vi "decimateInput.vi"(8 "reset":bool, 9 "input":i16, 10 "zeroOutput":bool, 11 "invert":bool) -> (3 "output":i16)   [LabVIEW 2016]
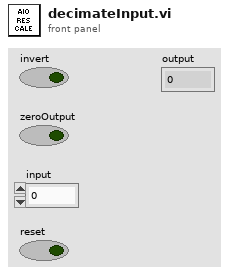
[diagram p1: front panel]
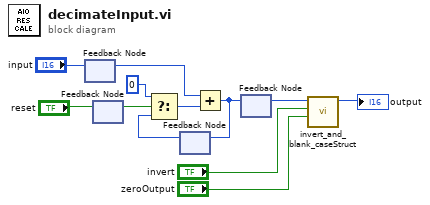
[diagram p0: block diagram]
diagram:
  n1 = feedback #1() -> (w11:i16)  [unwired: 1 in]
  n2 = feedback-in #1("input") -> ()
  n3 = feedback #2() -> (w9:bool)  [unwired: 1 in]
  n4 = feedback-in #2("reset") -> ()
  n5 = feedback #3() -> (w6:i16)  [unwired: 1 in]
  n6 = Select(t=i16 0, s=w9, f=w6) -> (s? t:f=w7:i16)
  n7 = Add(x=w11, y=w7) -> (x+y=w10:i16)
  n8 = feedback-in #3(w10) -> ()
  n9 = feedback #4() -> (w2:i16)  [unwired: 1 in]
  n10 = feedback-in #4(w10) -> ()
  n11 = call "invert_and_blank_caseStruct.vi"("zeroOutput"="zeroOutput", "invert"="invert", "input"=w2) -> ("output"=→"output":i16)  [unwired: 8 in]
